vi "Configure Frequency Characteristic.vi"(8 "error in (no error)":errorcluster, 9 "Frequency Unit (0: Frequency)":i32(ring) items=["Frequency", "Channel"], 10 "Enable Low Frequency Channel (F: Disable)":bool, 11 "VISA resource name":refnum<visa-resource-name>) -> (0 "error out":errorcluster, 3 "VISA resource name out":refnum<visa-resource-name>)   [LabVIEW 2022 SP3, in "Agilent N934X Series.lvlib"]
doc: "Configure the frequency settings.\n\nNote:\nThis VI is only applicable for N9321C, N9322C, N9323C, N9324C models."
uses:
  <instrlib>/Agilent N934X Series/Agilent N934X Series.lvlib
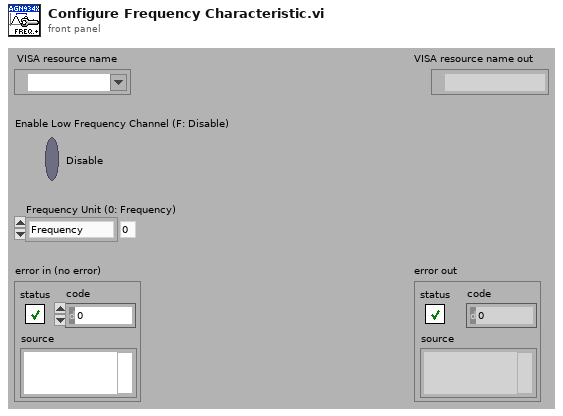
[diagram p1: front panel]
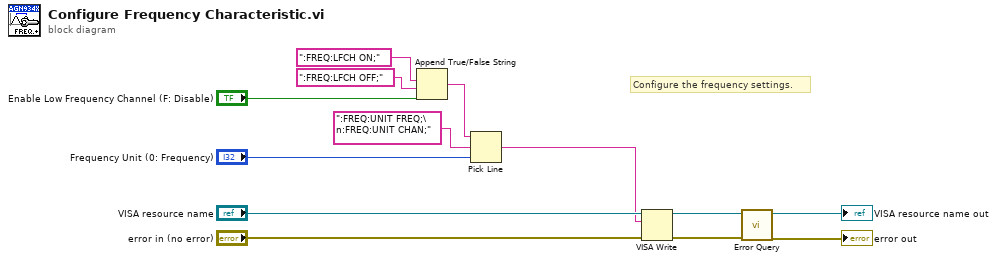
[diagram p0: block diagram]
diagram:
  # "Configure the frequency settings."
  n1 = Append True/False String(1:"Enable Low Frequency Channel (F: Disable)", 2:":FREQ:LFCH OFF;", 3:":FREQ:LFCH ON;") -> (0:w3:string)  [unwired: 1 in]
  n2 = Pick Line(string ("")=w3, multi-line string=":FREQ:UNIT FREQ;\n:FREQ:UNIT CHAN;", line index="Frequency Unit (0: Frequency)") -> (output string=w1:string)
  n3 = VISA Write(VISA resource name="VISA resource name", write buffer=w1, error in (no error)="error in (no error)") -> (VISA resource name out=w7:refnum<visa-resource-name>, error out=w6:errorcluster)  [unwired: 1 out]
  n4 = call <instrlib>:"Error Query.vi"("error in (no error)"=w6, "VISA resource name"=w7) -> ("error out"=→"error out":errorcluster, "VISA resource name out"=→"VISA resource name out":refnum<visa-resource-name>)  [unwired: 6 in, 2 out]
